vi "TDMS_Rx_read.vi"(0 "Array in":u64[](array[numeric]), 5 "PDW interpoter params":T3={"Fs (Hz)"=200000000.0, "fft size "=4096, "F base (Hz)"=2000000000.0, "min AMP (dB)"=0.0, "PW low bar (fft cycle)"=0.0, "Pw high bar (fft cycle)"=7000.0, "lo likege removal (fft bin)"=-1, "max gap (fft cycle)"=0.0}) -> (4 "Array":T2(array[cluster]), 8 "frequncy resolotion":dbl, 10 "PW_resolotion":dbl)   [LabVIEW 2021]
uses:
  fpga/vis/pulse detector/PDW interpoter params.ctl
panel:
  out "output cluster":T1
  in  "Cluster":T1
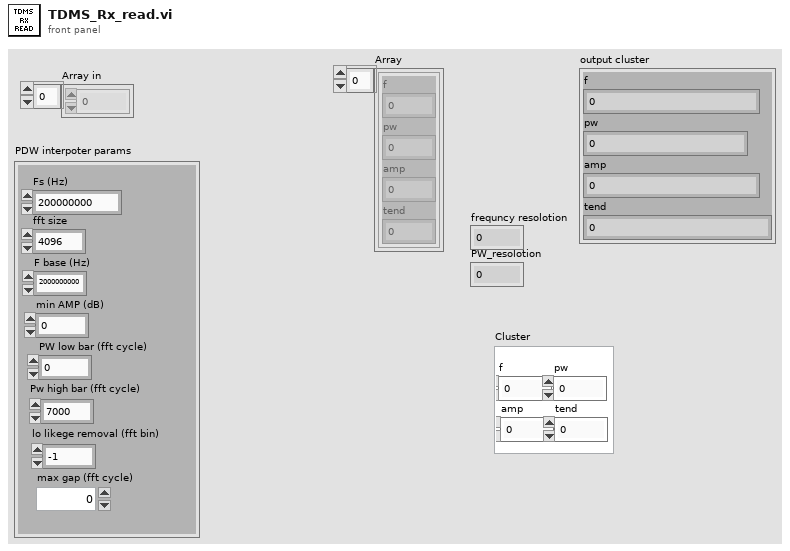
[diagram p1: front panel]
types:
  T1 = cluster{"f":dbl, "pw":dbl, "amp":dbl, "tend":dbl}
  T2 = cluster{"f":dbl, "pw":dbl, "amp":dbl, "tend":dbl}[]
  T3 = typedef "PDW interpoter params.ctl" = cluster{"Fs (Hz)":dbl, "fft size ":u32, "F base (Hz)":dbl, "min AMP (dB)":dbl, "PW low bar (fft cycle)":dbl, "Pw high bar (fft cycle)":dbl, "lo likege removal (fft bin)":i32, "max gap (fft cycle)":dbl}
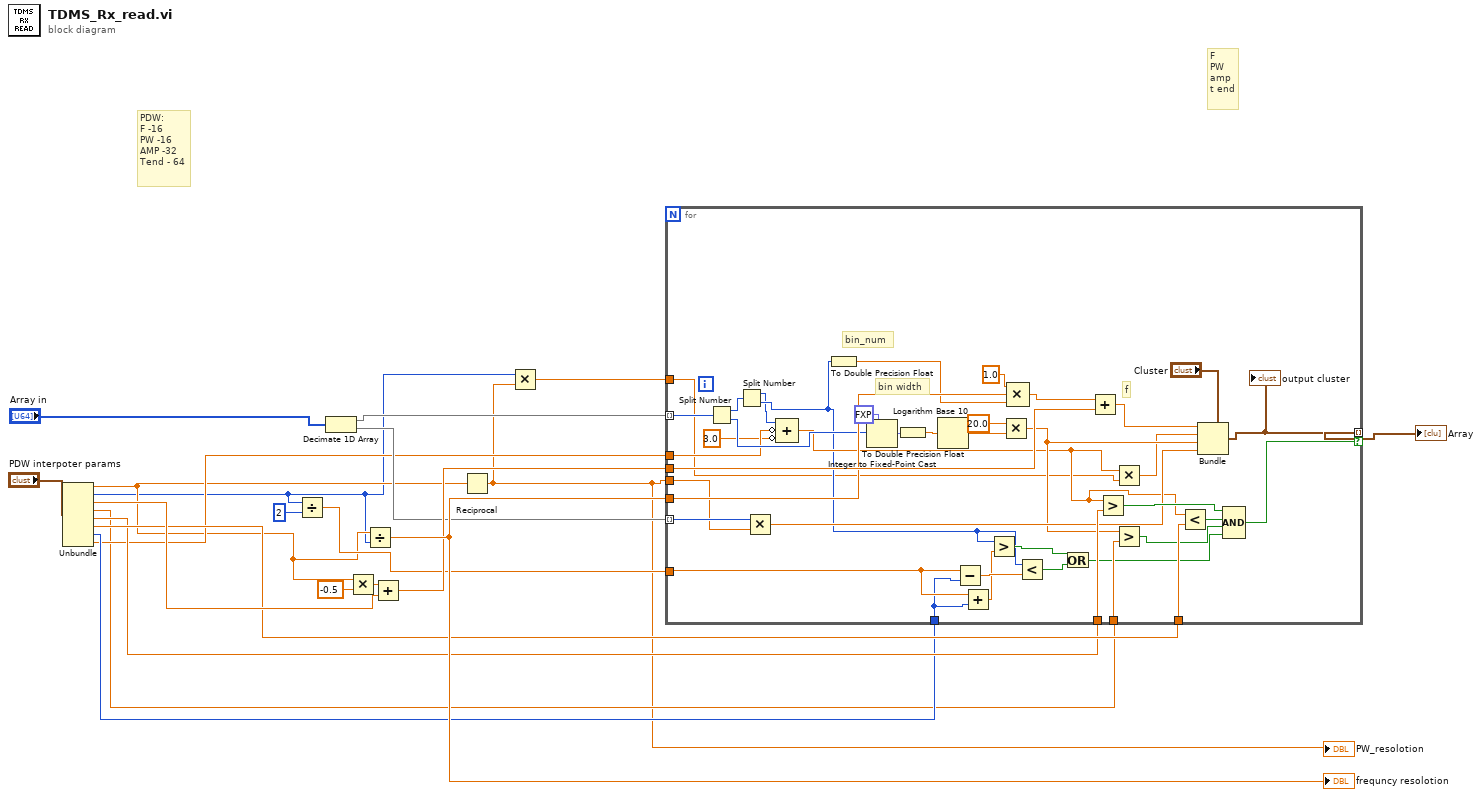
[diagram p0: block diagram]
diagram:
  # "F\nPW\namp\nt end"
  # "PDW:\nF -16\nPW -16\nAMP -32\nTend - 64"
  n1 = Unbundle("PDW interpoter params") -> ("Fs (Hz)"=w4:dbl, "fft size"=w3:u32, "F base (Hz)"=w12:dbl, "min AMP (dB)"=w7:dbl, "PW low bar (fft cycle)"=w10:dbl, "Pw high bar (fft cycle)"=w11:dbl, "lo likege removal (fft bin)"=w9:i32, "max gap (fft cycle)"=w8:dbl)
  n2 = Divide(x=w3, y=u32 2) -> (x/y=w5:dbl)
  n3 = Decimate 1D Array("Array in") -> (w16:u64[], w15:u64[])
  n4 = Multiply(x=w4, y=-0.5) -> (x*y=w19:dbl)
  n5 = Divide(x=w4, y=w3) -> (x/y=w21:dbl)
  "frequncy resolotion" <- w21
  n6 = Add(x=w19, y=w12) -> (x+y=w20:dbl)
  n7 = Reciprocal(x=w4) -> (1/x=w2:dbl)
  "PW_resolotion" <- w2
  n8 = Multiply(x=w3, y=w2) -> (x*y=w1:dbl)
  n9 = for {
    tunnel: w16 -> [w61] mode=indexing
    tunnel: w21 -> [w59]
    tunnel: w20 -> [w60]
    tunnel: [w57] -> w14 mode=indexing if=w29
    tunnel: w2 -> [w39]
    tunnel: w10 -> [w56]
    tunnel: w11 -> [w55]
    tunnel: w15 -> [w40] mode=indexing
    tunnel: w8 -> [w49]
    tunnel: w5 -> [w37]
    tunnel: w7 -> [w41]
    tunnel: w9 -> [w36]
    tunnel: w1 -> [w22]
    # "bin width"
    # "bin_num"
    # "f"
    n10 = Split Number(x=w61) -> (hi(x)=w62:u32, lo(x)=w53:u32)
    n11 = Split Number(x=w62) -> (hi(x)=w24:u16, lo(x)=w26:u16)
    n12 = Multiply(x=w40, y=w39) -> (x*y=w50:dbl)
    n13 = Compound Arithmetic op=unknown(w24, invert w49, invert 3.0 ("value")) -> (w28:dbl)
    n14 = To Double Precision Float(number=w26) -> (double precision float=w25:dbl)
    n15 = Integer to Fixed-Point Cast(fixed-point type=fxp<+/-,32,31> 0.0 ("fixed-point"), integer=w53) -> (fixed-point=w45:fxp<+/-,32,31>)
    n16 = To Double Precision Float(number=w45) -> (double precision float=w46:dbl)
    n17 = Logarithm Base 10(1:w46) -> (0:w44:dbl)
    n18 = Subtract(x=w37, y=w36) -> (x-y=w48:dbl)
    n19 = Add(x=w37, y=w36) -> (x+y=w35:dbl)
    n20 = Greater?(x=w26, y=w35) -> (0:w33:bool)
    n21 = Multiply(x=20.0, y=w44) -> (x*y=w43:dbl)
    n22 = Compound Arithmetic op=MULTIPLY(1.0 ("value"), w59, w25) -> (w27:dbl)
    n23 = Less?(x=w26, y=w48) -> (x < y?=w34:bool)
    n24 = Or(x=w33, y=w34) -> (x .or. y?=w32:bool)
    n25 = Add(x=w27, y=w60) -> (x+y=w58:dbl)
    n26 = Greater?(x=w28, y=w56) -> (0:w51:bool)
    n27 = Multiply(x=w28, y=w22) -> (x*y=w23:dbl)
    n28 = Greater?(x=w43, y=w41) -> (0:w31:bool)
    n29 = Less?(x=w28, y=w55) -> (x < y?=w54:bool)
    n30 = Bundle(cluster="Cluster", "f"=w58, "pw"=w23, "amp"=w43, "tend"=w50) -> (w57:T1)
    "output cluster" <- w57
    n31 = Compound Arithmetic op=AND(w51, w54, w31, w32) -> (w29:bool)
  }
  "Array" <- w14
